vi "Read Format string.vi"(8 "error in (no error)":errorcluster, 11 "Double D Element in":refnum<class "Double D Element.lvclass">) -> (0 "error out":errorcluster, 2 "Format string":string, 3 "Double D Element out":refnum<class "Double D Element.lvclass">)   [LabVIEW 2018, in "D Datagrid Library.lvlib" / "Double D Element.lvclass"]
uses:
  Double D Element.lvclass
  Floating point base/Floating point base.lvclass
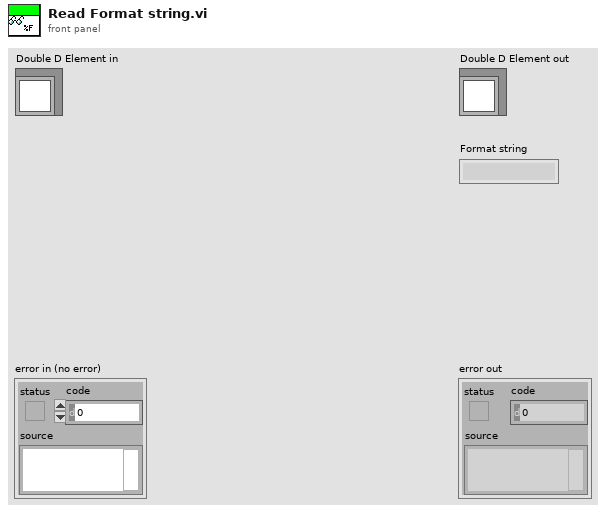
[diagram p1: front panel]
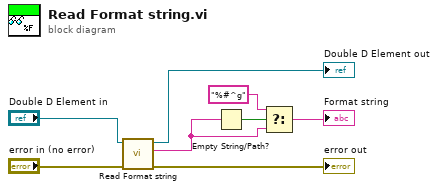
[diagram p0: block diagram]
diagram:
  n1 = call-parent "Read Format string.vi"("error in (no error)"="error in (no error)", "Floating point base in"="Double D Element in") -> ("error out"=→"error out":errorcluster, "Format string"=w2:string, "Floating point base out"=→"Double D Element out":refnum<class "Double D Element.lvclass">)  [unwired: 7 in]
  n2 = Empty String/Path?(string/path=w2) -> (empty?=w4:bool)
  n3 = Select(t="%#^g" ("format string"), s=w4, f=w2) -> (s? t:f=→"Format string":string)
